vi "error.From JSON String.vi"(8 "error in (no error)":errorcluster, 10 "JSON String":string, 11 "error in":refnum<class "error.lvclass">) -> (0 "error out":errorcluster, 3 "error out":refnum<class "error.lvclass">)   [LabVIEW 2020, in "JSON-RPC Lib.lvlib" / "error.lvclass"]
uses:
  error.lvclass
  Variant JSON API/Variant JSON API.lvlib
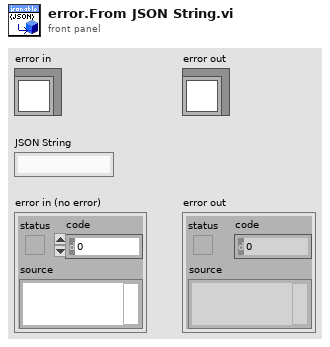
[diagram p1: front panel]
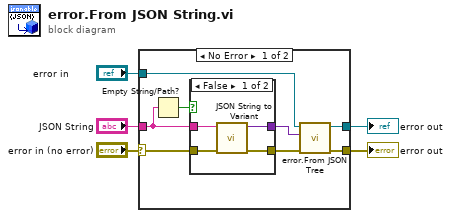
[diagram p0: block diagram]
diagram:
  n1 = case shown="No Error" "error in (no error)" {
    selector: "error in (no error)" -> [w10 w20]
    tunnel: [w11 w20] -> w4
    tunnel: [w12 w19] -> w2
    tunnel: "error in" -> [w13 w19]
    tunnel: "JSON String" -> [w8 _]
    frame No Error {
      n2 = Empty String/Path?(string/path=w8) -> (empty?=w7:bool)
      n3 = case shown="False" w7 {
        tunnel: w8 -> [w17 _]
        tunnel: [w16 _] -> w6
        tunnel: w10 -> [w14 w18]
        tunnel: [w15 w18] -> w9
        frame False {
          n4 = call "JSON String to Variant.vi"("error in (no error)"=w14, "JSON String"=w17) -> ("error out"=w15:errorcluster, "Variant out"=w16:variant)  [unwired: 8 in]
        }
        frame True {
        }
      }
      n5 = call "error.From JSON Tree.vi"("error in (no error)"=w9, "JSON Value in"=w6, "error in"=w13) -> (0:"error out"=w11:errorcluster, 3:"error out"=w12:refnum<class "error.lvclass">)  [unwired: 7 in]
    }
    frame Error {
    }
  }
  "error out" <- w4
  "error out" <- w2
